vi "okCFrontPanelDevices Get Device Serial Number.vi"(8 "Error In":errorcluster, 9 "Device ID":i32, 11 "okCFrontPanelDevices Refnum":refnum<k24>) -> (0 "Error Out":errorcluster, 1 "Serial Number":string, 3 "okCFrontPanelDevices Refnum":refnum<k24>)   [LabVIEW 2019, in "okFrontPanelC#Wrapper.lvlib"]
uses:
  okFrontPanelC#Wrapper.lvlib
  C:/UCLA Thinkpad Google Drive/LabVIEW 2019 SP1/builds/SS2 Live Distribution/Opal Kelly/C# Wrapper/libFrontPanel-csharp.dll
  libFrontPanel-csharp.dll
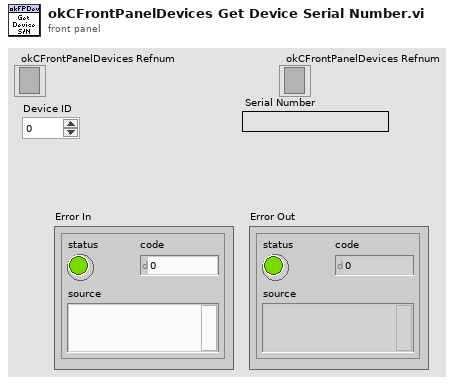
[diagram p1: front panel]
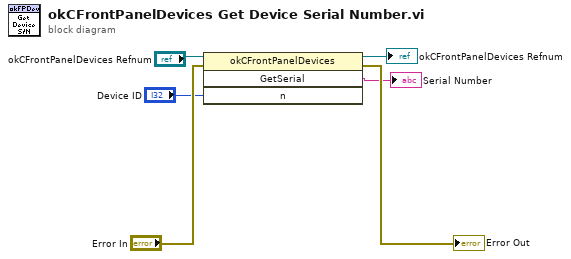
[diagram p0: block diagram]
diagram:
  n1 = invoke class="okCFrontPanelDevices" method="GetSerial"(reference="okCFrontPanelDevices Refnum", error in="Error In", "n"="Device ID") -> (reference out=→"okCFrontPanelDevices Refnum":refnum<k24>, error out=→"Error Out":errorcluster, "GetSerial"=→"Serial Number":string)  [unwired: 1 in, 1 out]
